vi "Stop Core.vi"(10 "final error code":i32, 11 "Main_Control in":refnum<class "Main_Control.lvclass">) -> (3 "Main_Control out":refnum<class "Main_Control.lvclass">)   [LabVIEW 2021, in "Main_Control.lvlib" / "Main_Control.lvclass"]
doc: "(<B>Filename</B>: Actor Framework.lvlib:Actor.lvclass:Stop Core.vi)\n\nDefines what the actor does before it stops. Use the <B>final error code</B> input to determine whether the actor shut down in response to an error.\n\nBy default, this method does nothing. A descendant class may override it to define behavior, such as shutting down any processes the actor initiated in its override of the Actor Core method."
uses:
  Main_Control.lvclass
  Main_Control.lvclass/Main_Control.ctl
  <vilib>/ActorFramework/Actor/Actor.lvclass
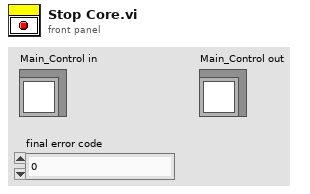
[diagram p1: front panel]
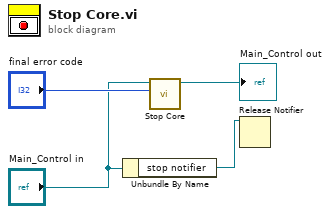
[diagram p0: block diagram]
diagram:
  n1 = Unbundle By Name("Main_Control in") -> ("stop notifier"=w1:refnum<notifier>)
  n2 = call-parent "Stop Core.vi"("final error code"="final error code", "Actor in"="Main_Control in") -> ("Actor out"=→"Main_Control out":refnum<class "Main_Control.lvclass">)  [unwired: 9 in]
  n3 = Release Notifier(notifier=w1) -> ()  [unwired: 2 in, 3 out]
